vi "Get Path.vi"(0 "GMaps API in":refnum<class "GMaps API.lvclass">, 5 "error in (no error)":errorcluster) -> (14 "GMaps API out":refnum<class "GMaps API.lvclass">, 15 "Concatenated Path":string, 19 "error out":errorcluster)   [LabVIEW 2016, in "GMaps API.lvclass"]
doc: "Gets a set of one or more locations connected by a path to overlay on the map image."
uses:
  GMaps API.lvclass
  GMaps API.lvclass/GMaps API.ctl
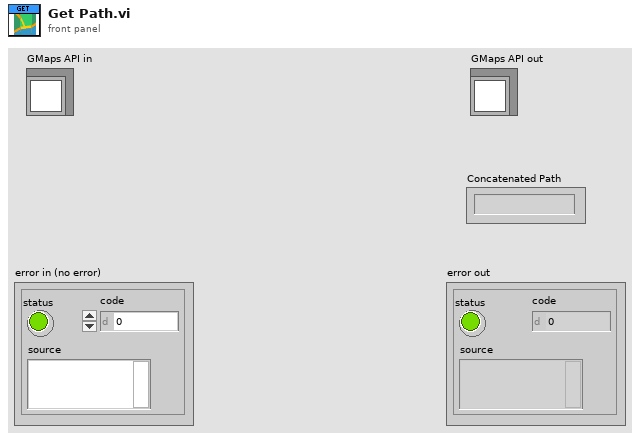
[diagram p1: front panel]
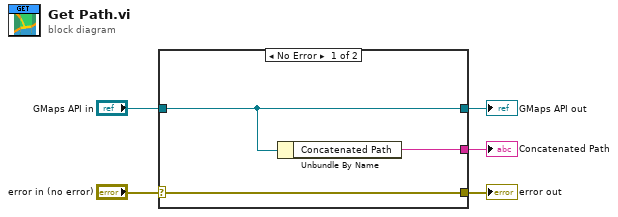
[diagram p0: block diagram]
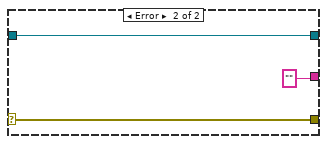
[diagram p2: hidden frame]
diagram:
  n1 = case shown="No Error" "error in (no error)" {
    selector: "error in (no error)" -> [w8 w11]
    tunnel: [w8 w11] -> w4
    tunnel: [w7 w10] -> w2
    tunnel: "GMaps API in" -> [w7 w10]
    tunnel: [w6 ""] -> w1
    frame No Error {
      n2 = Unbundle By Name(w7) -> ("Concatenated Path"=w6:string)
    }
    frame Error {
    }
  }
  "error out" <- w4
  "GMaps API out" <- w2
  "Concatenated Path" <- w1
